vi "Actor Core.vi"(8 "error in":errorcluster, 11 "Nested in":refnum<class "UI.lvclass">) -> (0 "error out":errorcluster, 3 "Actor out":refnum<class "Actor.lvclass">)   [LabVIEW 2020, in "UI.lvlib" / "UI.lvclass"]
doc: "(<B>Filename</B>: Actor Framework.lvlib:Actor.lvclass:Actor Core.vi)\n\nReceives messages to the actor, reacts to them, and initiates any error handling that may shut the actor down.\n\nDescendant classes may override this VI to append parallel tasks for the actor to complete while it handles messages. Overrides use the Call Parent Method node."
uses:
  UI.lvclass
  C:/Program Files (x86)/National Instruments/LabVIEW 2020/vi.lib/ActorFramework/Actor/Actor.lvclass
  <vilib>/ActorFramework/Actor/Actor.lvclass
  Turnos/Turnos.lvclass
  Paquetes/Paquetes.lvclass
  Dinero/Dinero.lvclass
  UI.lvclass/UI.ctl
  Turnos/Turnos.lvclass/Turnos.ctl
  Paquetes/Paquetes.lvclass/Paquetes.ctl
  Dinero/Dinero.lvclass/Dinero.ctl
  <vilib>/ActorFramework/Actor/Actor.lvclass/Actor.ctl
  <vilib>/ActorFramework/Message Enqueuer/Message Enqueuer.lvclass/Message Enqueuer.ctl
  <vilib>/ActorFramework/Message Enqueuer/Init from Existing Queue.vi
  <vilib>/ActorFramework/Message Enqueuer/Enqueue.vi
  <vilib>/ActorFramework/Stop Msg/Stop Msg.lvclass
  C:/Program Files (x86)/National Instruments/LabVIEW 2020/vi.lib/ActorFramework/Message/Message.lvclass
  <vilib>/ActorFramework/Message Priority Queue/Priority Enqueue.vi
  <vilib>/ActorFramework/Message Enqueuer/Message Enqueuer.lvclass
  C:/Users/HP/Desktop/Salma_Aguayo/UI/UI.lvclass
  C:/Users/HP/Desktop/Salma_Aguayo/Turnos/Turnos.lvclass
  C:/Users/HP/Desktop/Salma_Aguayo/Paquetes/Paquetes.lvclass
  C:/Users/HP/Desktop/Salma_Aguayo/Dinero/Dinero.lvclass
panel:
  out "SERIVICIO":string
  out "Cambio":i32
  out "Credito":i32
  in  "Contabilidad":bool
  in  "Stop Total":bool
  in  "Stop":bool
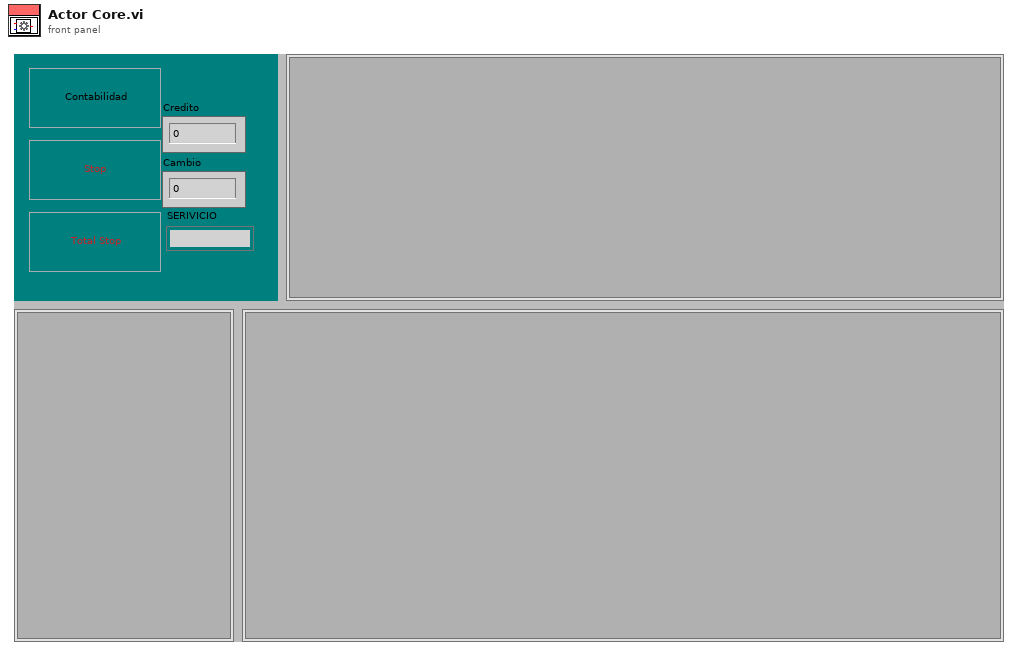
[diagram p1: front panel]
types:
  T1 = cluster{"Stop":refnum<user-event>, "Credito":refnum<user-event>, "Cambio":refnum<user-event>, "SERIVICIO":refnum<user-event>}
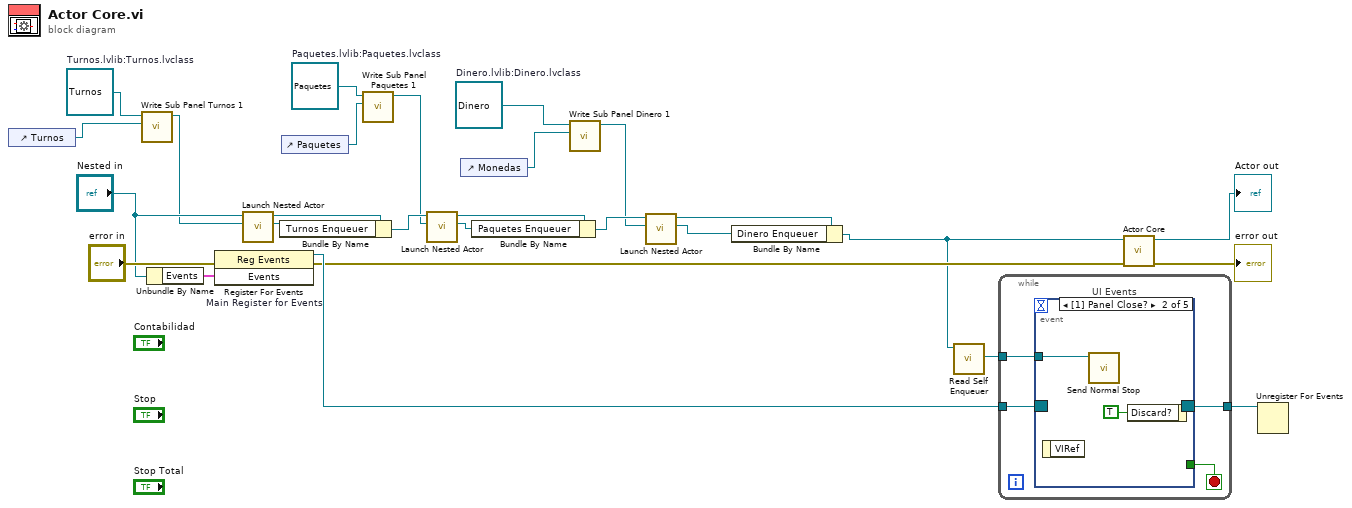
[diagram p0: block diagram]
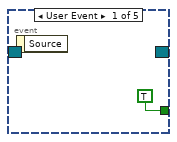
[diagram p2: hidden frame]
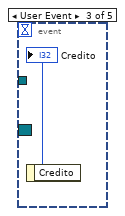
[diagram p3: hidden frame]
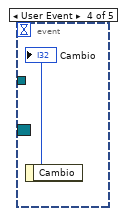
[diagram p4: hidden frame]
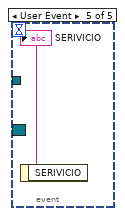
[diagram p5: hidden frame]
diagram:
  w6 = refnum<class "Dinero.lvclass"> refnum  # Dinero.lvlib:Dinero.lvclass
  w13 = refnum<class "Paquetes.lvclass"> refnum  # Paquetes.lvlib:Paquetes.lvclass
  w19 = refnum<class "Turnos.lvclass"> refnum  # Turnos.lvlib:Turnos.lvclass
  n1 = control-ref of="Turnos"() -> (w17:refnum<vi>)
  n2 = call "Write Sub Panel Turnos 1.vi"("Sub Panel Turnos"=w17, "Turnos in"=w19) -> ("Turnos out"=w16:refnum<class "Turnos.lvclass">)  [unwired: 8 in, 1 out]
  n3 = Unbundle By Name("Nested in") -> ("Events"=w24:T1)
  n4 = register-events "Main Register for Events"(error in="error in", w24) -> (reference out=w25:refnum<event-registration>, error out=w20:errorcluster)  [unwired: 1 in]
  n5 = call <vilib>:"Launch Nested Actor.vi"("Nested Actor"=w16, "Caller Actor in"="Nested in") -> ("Nested Actor's Enqueuer"=w14:refnum<class "Message Enqueuer.lvclass">, "Caller Actor out"=w15:refnum<class "UI.lvclass">)  [unwired: 7 in, 1 out]
  n6 = Bundle By Name(cluster=w15, "Turnos Enqueuer"=w14) -> (w11:refnum<class "UI.lvclass">)
  n7 = control-ref of="Paquetes"() -> (w12:refnum<vi>)
  n8 = call "Write Sub Panel Paquetes 1.vi"("Sub Panel Paquetes"=w12, "Paquetes in"=w13) -> ("Paquetes out"=w10:refnum<class "Paquetes.lvclass">)  [unwired: 8 in, 1 out]
  n9 = call <vilib>:"Launch Nested Actor.vi"("Nested Actor"=w10, "Caller Actor in"=w11) -> ("Nested Actor's Enqueuer"=w8:refnum<class "Message Enqueuer.lvclass">, "Caller Actor out"=w9:refnum<class "UI.lvclass">)  [unwired: 7 in, 1 out]
  n10 = control-ref of="Monedas"() -> (w5:refnum<vi>)
  n11 = Bundle By Name(cluster=w9, "Paquetes Enqueuer"=w8) -> (w7:refnum<class "UI.lvclass">)
  n12 = call "Write Sub Panel Dinero 1.vi"("Sub Panel Dinero"=w5, "Dinero in"=w6) -> ("Dinero out"=w4:refnum<class "Dinero.lvclass">)  [unwired: 8 in, 1 out]
  n13 = call <vilib>:"Launch Nested Actor.vi"("Nested Actor"=w4, "Caller Actor in"=w7) -> ("Nested Actor's Enqueuer"=w2:refnum<class "Message Enqueuer.lvclass">, "Caller Actor out"=w3:refnum<class "UI.lvclass">)  [unwired: 7 in, 1 out]
  n14 = Bundle By Name(cluster=w3, "Dinero Enqueuer"=w2) -> (w1:refnum<class "UI.lvclass">)
  n15 = call <vilib>:"Read Self Enqueuer.vi"("Actor"=w1) -> ("Self Enqueuer"=w22:refnum<class "Message Enqueuer.lvclass">)  [unwired: 10 in]
  n16 = while {
    tunnel: w25 -> [w31]
    tunnel: [w29] -> w23
    tunnel: w22 -> [w28]
    stop <- w30 stop-if-true
    n17 = event "UI Events" shown="[1] Panel Close?" {
      selector: w31 -> [_ _ _ _ _]
      dyn-events: [_ _ _ _ _] -> w29
      timeout: _ -> [_ _ _ _ _]
      tunnel: [TRUE _ _ _ _] -> w30
      tunnel: w28 -> [_ w33 _ _ _]
      event User Event {
        n18 = event-data() -> ()  [unwired: 1 in, 1 out]
      }
      event Panel Close? {
        n19 = event-data() -> ()  [unwired: 1 in, 1 out]
        n20 = call <vilib>:"Send Normal Stop.vi"("Message Enqueuer"=w33) -> ()  [unwired: 10 in, 1 out]
        n21 = event-data("Discard?"=TRUE) -> ()  [unwired: 1 in, 1 out]
      }
      event User Event {
        n22 = event-data() -> ("Credito"=→"Credito":i32)  [unwired: 1 in]
      }
      event User Event {
        n23 = event-data() -> ("Cambio"=→"Cambio":i32)  [unwired: 1 in]
      }
      event User Event {
        n24 = event-data() -> ("SERIVICIO"=→"SERIVICIO":string)  [unwired: 1 in]
      }
    }
  }
  n25 = call-parent "Actor Core.vi"("error in"=w20, "Actor in"=w1) -> ("error out"=→"error out":errorcluster, "Actor out"=→"Actor out":refnum<class "Actor.lvclass">)  [unwired: 8 in]
  n26 = Unregister For Events(event registration refnum=w23) -> ()  [unwired: 1 in, 1 out]
